vi "Get Greeter_req.vi"(8 "error in (no error)":errorcluster, 11 "gRPCid":T1) -> (0 "error out":errorcluster, 2 "package_templatemessage":T2, 3 "gRPCid out":T1)   [LabVIEW 2019, in "Generated_server.lvlib"]
uses:
  Generated_server.lvlib
  Greeter_req.ctl
  Greeter_req_req_oneof/Greeter_req_req_oneof.lvclass
  <vilib>/gRPC/LabVIEW gRPC Library/Shared/grpcId.ctl
  Greeter_req_Flat.ctl
  Greeter_req_req_oneof/Greeter_req_req_oneof.lvclass/Greeter_req_req_oneof.ctl
  2ed25e12-861d-4677-8ead-ace2906b2041.vi
  <vilib>/gRPC/LabVIEW gRPC Library/Shared/TranslateGrpcError.vi
  Greeter_req_req_oneof/Setreq_int32.vi
  Greeter_req_req_oneof/Setreq_int64.vi
  Greeter_req_req_oneof/Setreq_uint32.vi
  Greeter_req_req_oneof/Setreq_uint64.vi
  Greeter_req_req_oneof/Setreq_sint32.vi
  Greeter_req_req_oneof/Setreq_sint64.vi
  Greeter_req_req_oneof/Setreq_fixed32.vi
  Greeter_req_req_oneof/Setreq_fixed64.vi
  Greeter_req_req_oneof/Setreq_sfixed32.vi
  Greeter_req_req_oneof/Setreq_sfixed64.vi
  Greeter_req_req_oneof/Setreq_float.vi
  Greeter_req_req_oneof/Setreq_double.vi
  Greeter_req_req_oneof/Setreq_bool.vi
  Greeter_req_req_oneof/Setreq_string.vi
  Greeter_req_req_oneof/Setreq_bytes.vi
  <vilib>/gRPC/LabVIEW gRPC Library/Server API/Server/Get Server DLL Path.vi
  <vilib>/Utility/error.llb/Error Cluster From Error Code.vi
  <vilib>/Utility/error.llb/Simple Error Handler.vi
  Greeter_req_req_oneof/GetFieldFromProtobufIndexGreeter_req_req_oneof.vi
  <vilib>/gRPC/LabVIEW gRPC Library/grpc-lvsupport-release.lvlib
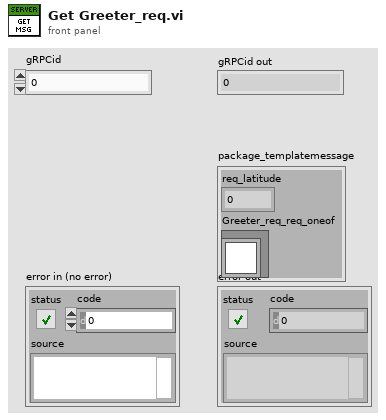
[diagram p1: front panel]
types:
  T1 = typedef "grpc-lvsupport-release.lvlib/grpcId.ctl" = u64
  T2 = typedef "Generated_server.lvlib/Greeter_req.ctl" = cluster{"req_latitude":i32, "Greeter_req_req_oneof":refnum<class "Greeter_req_req_oneof.lvclass">}
  T3 = typedef "Generated_server.lvlib/Greeter_req_Flat.ctl" = cluster{"req_latitude":i32, "Greeter_req_req_oneof_selected_index":i32, "req_int32":i32, "req_int64":i64, "req_uint32":u32, "req_uint64":u64, "req_sint32":i32, "req_sint64":i64, "req_fixed32":u32, "req_fixed64":u64, "req_sfixed32":i32, "req_sfixed64":i64, "req_float":sgl, "req_double":dbl, "req_bool":bool, "req_string":string, "req_bytes":u8[]}
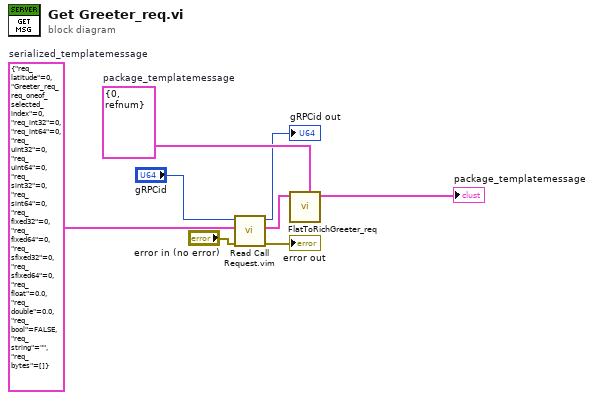
[diagram p0: block diagram]
diagram:
  w6 = T3 {"req_latitude"=0, "Greeter_req_req_oneof_selected_index"=0, "req_int32"=0, "req_int64"=0, "req_uint32"=0, "req_uint64"=0, "req_sint32"=0, "req_sint64"=0, "req_fixed32"=0, "req_fixed64"=0, "req_sfixed32"=0, "req_sfixed64"=0, "req_float"=0.0, "req_double"=0.0, "req_bool"=FALSE, "req_string"="", "req_bytes"=[]}  # serialized_templatemessage
  w5 = T2 {"req_latitude"=0, "Greeter_req_req_oneof"=refnum}  # package_templatemessage
  n1 = call "Read Call Request.vim"("error in"="error in (no error)", "Request Type"=w6, "gRPCid in"="gRPCid") -> ("error out"=→"error out":errorcluster, "Request Data"=w4:T3, "gRPCid out"=→"gRPCid out":T1)  [unwired: 6 in]
  n2 = call "FlatToRichGreeter_req.vi"("OutputClusterType"=w5, "InputCluster"=w4) -> ("OutputCluster"=→"package_templatemessage":T2)  [unwired: 9 in]
